vi "Image2Array.vi"(8 "error in (no error)":errorcluster, 10 "Image Type":T1 items=["Grayscale (U8)", "Grayscale (I16)", "Grayscale (SGL)", "Complex (CSG)", "RGB (U32)", "HSL (U32)", "RGB (U64)", "Grayscale (U16)"], 11 "Image":T2) -> (0 "error out":errorcluster, 3 "Image Pixels (U32)":u32[][](array[numeric]))   [LabVIEW 2017, in "ImageAcquisitionLibrary.lvlib"]
uses:
  <vilib>/vision/Image Controls.llb/IMAQ Image.ctl
  ImageAcquisitionLibrary.lvlib
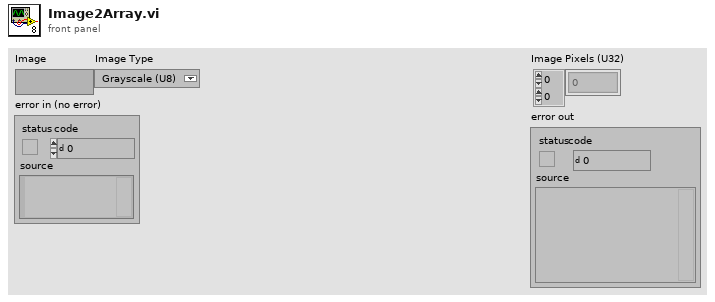
[diagram p1: front panel]
types:
  T1 = typedef "Image Type" = u32
  T2 = typedef "IMAQ Image.ctl" = refnum<image>
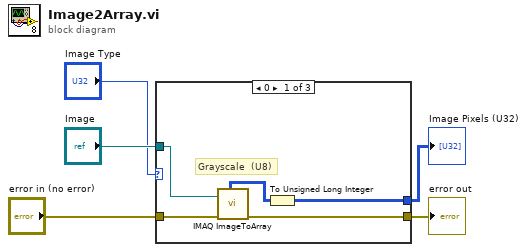
[diagram p0: block diagram]
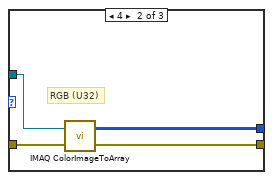
[diagram p2: hidden frame]
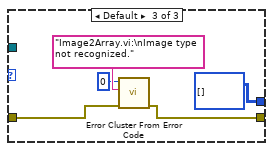
[diagram p3: hidden frame]
diagram:
  n1 = case shown="0" "Image Type" {
    tunnel: "Image" -> [w9 w14 _]
    tunnel: "error in (no error)" -> [w8 w13 w18]
    tunnel: [w7 w12 w17] -> w4
    tunnel: [w10 w11 u32[][] [] ("Image Pixels (U32)")] -> w3
    frame 0 {
      # "Grayscale  (U8)"
      n2 = call "IMAQ ImageToArray"("error in (no error)"=w8, "Image"=w9) -> ("error out"=w7:errorcluster, "Image Pixels (U8)"=w6:u8[][])  [unwired: 2 in, 3 out]
      n3 = To Unsigned Long Integer(number=w6) -> (unsigned 32bit integer=w10:u32[][])
    }
    frame 4 {
      # "RGB (U32)"
      n4 = call "IMAQ ColorImageToArray"("Image"=w14, "error in (no error)"=w13) -> ("Image Pixels (U32)"=w11:u32[][], "error out"=w12:errorcluster)  [unwired: 2 in, 1 out]
    }
    frame Default {
      n5 = call <vilib>:"Error Cluster From Error Code.vi"("error in (no error)"=w18, "error message (\"\")"="Image2Array.vi:\nImage type not recognized." ("error message (\"\")"), "error code (0)"=0) -> ("error out"=w17:errorcluster)  [unwired: 6 in]
    }
  }
  "error out" <- w4
  "Image Pixels (U32)" <- w3
